vi "WriteLeftSubpanel.vi"(8 "error in (no error)":errorcluster, 10 "Left Subpanel":refnum<vi>, 11 "EmbeddedMainUI in":refnum<class "EmbeddedMainUI.lvclass">) -> (0 "error out":errorcluster, 3 "EmbeddedMainUI out":refnum<class "EmbeddedMainUI.lvclass">)   [LabVIEW 2016, in "EmbeddedMainUI.lvclass"]
uses:
  EmbeddedMainUI.lvclass
  EmbeddedMainUI.lvclass/EmbeddedMainUI.ctl
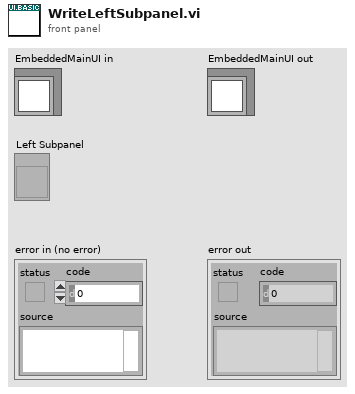
[diagram p1: front panel]
types:
  T1 = typedef "EmbeddedMainUI.lvclass/FrameworkDataRef.ctl" = refnum<data-value>
  T2 = typedef "EmbeddedMainUI.lvclass/FrameworkData.ctl" = cluster{"Subpanels":refnum<class "EmbeddedSMO.lvclass">[], "Left Subpanel":refnum<vi>, "Right Subpanel":refnum<vi>, "Active Left":i32, "Active Right":i32}
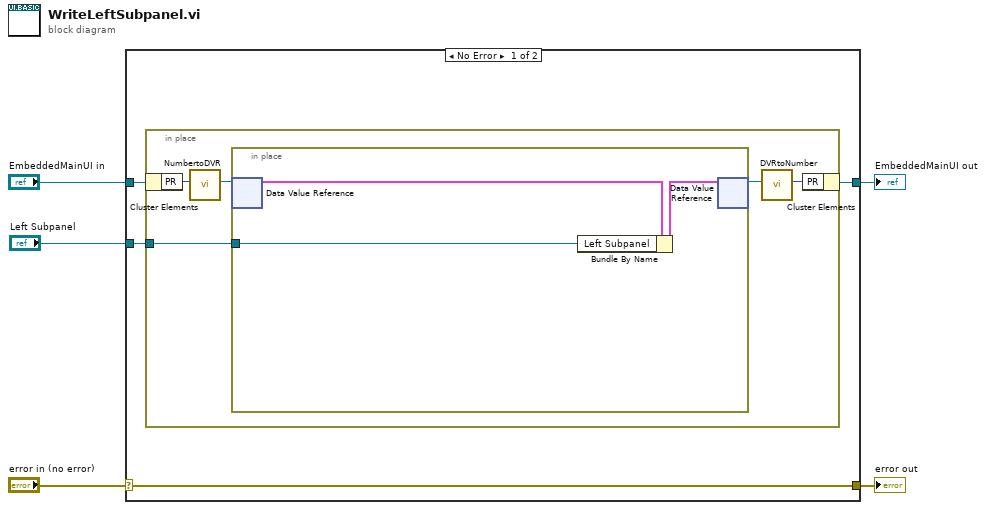
[diagram p0: block diagram]
diagram:
  n1 = case shown="No Error" "error in (no error)" {
    selector: "error in (no error)" -> [w9 w19]
    tunnel: [w9 w19] -> w4
    tunnel: [w7 w18] -> w2
    tunnel: "EmbeddedMainUI in" -> [w8 w18]
    tunnel: "Left Subpanel" -> [w6 _]
    frame No Error {
      n2 = in-place {
        in-place-border: w6 -> [w10]
        n3 = in-place-cluster #1(w8) -> ("PR"=w14:i32)
        n4 = call "NumbertoDVR.vi"("Numeric"=w14) -> ("FrameworkDataRef"=w12:T1)  [unwired: 10 in]
        n5 = in-place {
          in-place-border: w10 -> [w15]
          n6 = in-place-dvr #2(w12) -> (w17:T2)  [unwired: 1 out]
          n7 = Bundle By Name(cluster=w17, "Left Subpanel"=w15) -> (w16:T2)
          n8 = in-place-dvr #2(w16) -> (w11:T1)  [unwired: 1 out]
        }
        n9 = call "DVRtoNumber.vi"("FrameworkDataRef"=w11) -> ("Number"=w13:i32)  [unwired: 10 in]
        n10 = in-place-cluster #1("PR"=w13) -> (w7:refnum<class "EmbeddedMainUI.lvclass">)
      }
    }
    frame Error {
    }
  }
  "error out" <- w4
  "EmbeddedMainUI out" <- w2
